vi "Get Parent Library.vi"(8 "error in (no error)":errorcluster, 11 "Library in":refnum<vi>) -> (0 "error out":errorcluster, 2 "Parent Library":refnum<vi>, 3 "Library out":refnum<vi>)   [LabVIEW 2015, in "UniquifyFullyQualifiedVIName.lvclass"]
uses:
  UniquifyFullyQualifiedVIName.lvclass
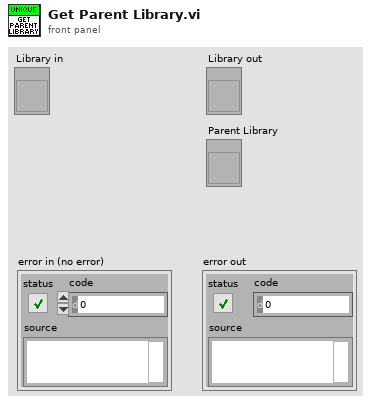
[diagram p1: front panel]
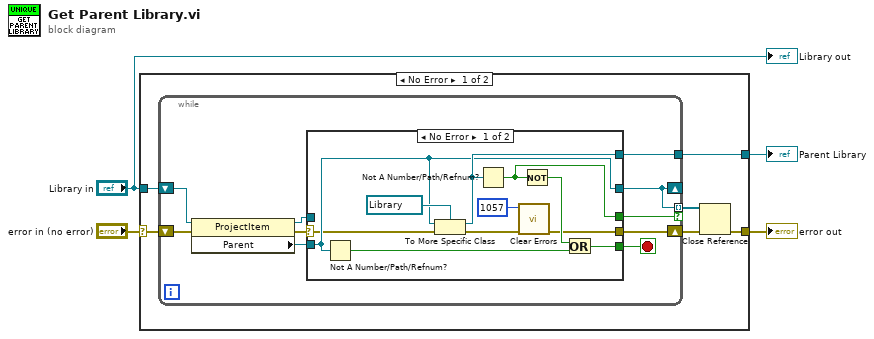
[diagram p0: block diagram]
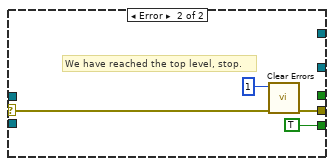
[diagram p2: hidden frame]
diagram:
  n1 = case shown="No Error" "error in (no error)" {
    selector: "error in (no error)" -> [w9 w36]
    tunnel: [w10 _] -> w4
    tunnel: [w6 w36] -> w3
    tunnel: "Library in" -> [w8 _]
    frame No Error {
      n2 = while {
        shift-right: [w17] -> _
        shift-left: w8 -> [w13]
        tunnel: [w19] -> w10
        shift-right: [w18] -> w7
        shift-left: w9 -> [w15]
        tunnel: [w17] -> w5 mode=indexing if=w16
        stop <- w20 stop-if-true
        n3 = property class="ProjectItem"(reference=w13, error in=w15) -> (reference out=w12:refnum<vi>, error out=w14:errorcluster, "Parent"=w11:refnum<vi>)
        n4 = case shown="No Error" w14 {
          selector: w14 -> [w21 w33]
          tunnel: [w26 TRUE] -> w20
          tunnel: [w25 _] -> w19
          tunnel: [w24 w32] -> w18
          tunnel: [w22 _] -> w17
          tunnel: [w23 _] -> w16
          tunnel: w12 -> [_ _]
          tunnel: w11 -> [w22 _]
          frame No Error {
            n5 = Not A Number/Path/Refnum?(number/path/refnum=w22) -> (NaN/Path/Refnum?=w27:bool)
            n6 = To More Specific Class(target class=refnum<vi> refnum ("reference"), reference=w22, error in=w21) -> (specific class reference=w25:refnum<vi>, error out=w31:errorcluster)
            n7 = Not A Number/Path/Refnum?(number/path/refnum=w25) -> (NaN/Path/Refnum?=w23:bool)
            n8 = call <vilib>:"Clear Errors.vi"("error in (no error)"=w31, "specific error code to clear (0: all)"=1057) -> ("error out"=w24:errorcluster)  [unwired: 4 in, 1 out]
            n9 = Not(x=w23) -> (.not. x?=w28:bool)
            n10 = Or(x=w28, y=w27) -> (x .or. y?=w26:bool)
          }
          frame Error {
            # "We have reached the top level, stop."
            n11 = call <vilib>:"Clear Errors.vi"("error in (no error)"=w33, "specific error code to clear (0: all)"=1) -> ("error out"=w32:errorcluster)  [unwired: 4 in, 1 out]
          }
        }
      }
      n12 = Close Reference(reference=w5, error in (no error)=w7) -> (error out=w6:errorcluster)
    }
    frame Error {
    }
  }
  "Parent Library" <- w4
  "error out" <- w3
  "Library out" <- "Library in"
